vi "Compute Branch Rate.vi"(8 "error in (no error)":errorcluster, 11 "Coverage in":refnum<class "Coverage.lvclass">) -> (0 "error out":errorcluster, 3 "Coverage out":refnum<class "Coverage.lvclass">)   [LabVIEW 2017, in "Cobertura.lvlib" / "Coverage.lvclass"]
uses:
  Coverage.lvclass
  Coverage.lvclass/Coverage.ctl
  Package/Package.lvclass/Package.ctl
  Package/Read Branch Rate.vi
  Package/Package.lvclass
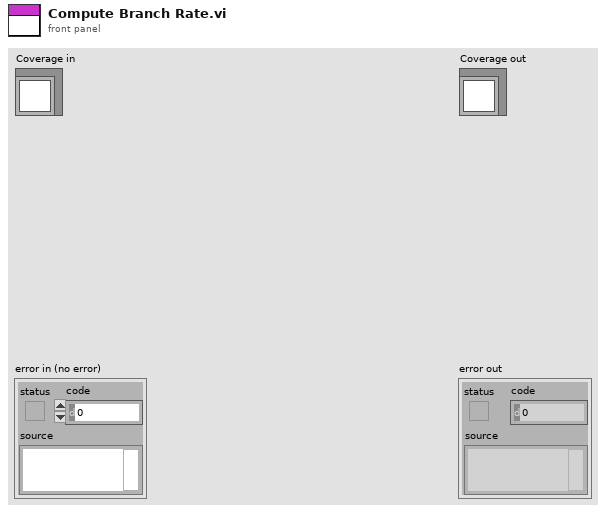
[diagram p1: front panel]
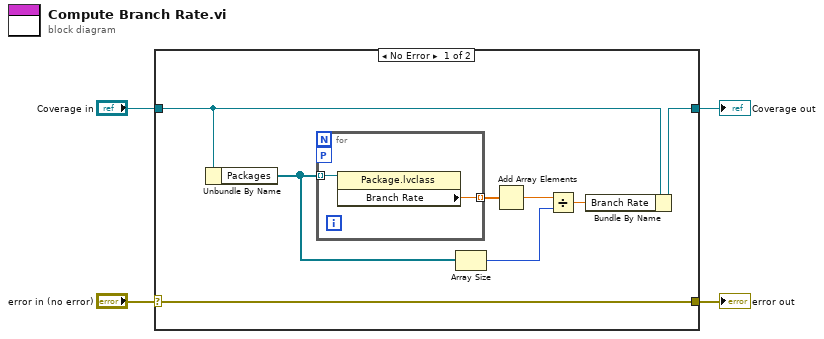
[diagram p0: block diagram]
diagram:
  n1 = case shown="No Error" "error in (no error)" {
    selector: "error in (no error)" -> [w12 w16]
    tunnel: [w12 w16] -> w3
    tunnel: [w5 w15] -> w1
    tunnel: "Coverage in" -> [w6 w15]
    frame No Error {
      n2 = Unbundle By Name(w6) -> ("Packages"=w9:refnum<class "Package.lvclass">[])
      n3 = for {
        tunnel: w9 -> [w14] mode=indexing
        tunnel: [w13] -> w11 mode=indexing
        workers-P: _ -> [_]
        n4 = property class="Package.lvclass"(reference=w14) -> ("Branch Rate"=w13:dbl)  [unwired: 1 in, 2 out]
      }
      n5 = Array Size(array=w9) -> (size(s)=w8:i32)
      n6 = Add Array Elements(numeric array=w11) -> (sum=w10:dbl)
      n7 = Divide(x=w10, y=w8) -> (x/y=w7:dbl)
      n8 = Bundle By Name(cluster=w6, "Branch Rate"=w7) -> (w5:refnum<class "Coverage.lvclass">)
    }
    frame Error {
    }
  }
  "error out" <- w3
  "Coverage out" <- w1
